vi "Host Main.vi"() -> ()   [LabVIEW 2015]
doc: "This application launches and executes the Tag Bus Data framework configuration for the specified target alias. This is a simple example of the framework API functions, but may also be a suitable starting point for a Host UI or Thick Client that is running a local version of the framework."
uses:
  <vilib>/NI/Module Execution Interface/Engine Runtime/Execution States.ctl
  <vilib>/NI/Module Execution Interface/Engine Runtime/Fault.ctl
  <vilib>/NI/Tag Bus Module Framework/runtime/error classification.ctl
  <vilib>/NI/Current Value Table/DataTypes/Double_Read.vi
  <vilib>/NI/Current Value Table/Type to Enum.vi
  <vilib>/NI/Current Value Table/DataTypes/Double_Type To Enum.vi
  <vilib>/NI/Current Value Table/FGVs/CVT Globals.vi
  <vilib>/NI/Current Value Table/FGVs/Tag Memory.vi
  <vilib>/NI/Current Value Table/Memory Block.vi
  <vilib>/NI/Current Value Table/DataTypes/Double_Memory Block.vi
  <vilib>/NI/Module Execution Interface/Engine Runtime/Engine Runtime Interface.lvclass
  <vilib>/NI/DCAF/Tag Editor Core/Framework Configuration Classes/target runtime/PL_Target Runtime.lvclass
  <vilib>/NI/Tag Bus Module Framework/FPGA manager/FPGA manager.lvlib
  <vilib>/rvi/interface/nirviOpenFPGA/nirviOpenFPGA.xnode
  <vilib>/userdefined/High Color/nirio_resource_hc.ctl
  <vilib>/NI/Tag Bus Module Framework/FPGA manager/methods.ctl
  <vilib>/NI/Tag Bus Module Framework/runtime/TBM module execution interface.lvclass
  <vilib>/NI/Current Value Table/Current Value Table.lvlib
panel:
  out "Temperature":dbl
  in  "configuration file path":path=path "C:/Users/blueuser/Desktop/Hands On/Hands-On_1/myExercises/Temperature Controller/SimulatedSystem.pcfg"
  in  "target alias":string="PC"
  out "engine status":T4(array[cluster])
  in  "stop":bool
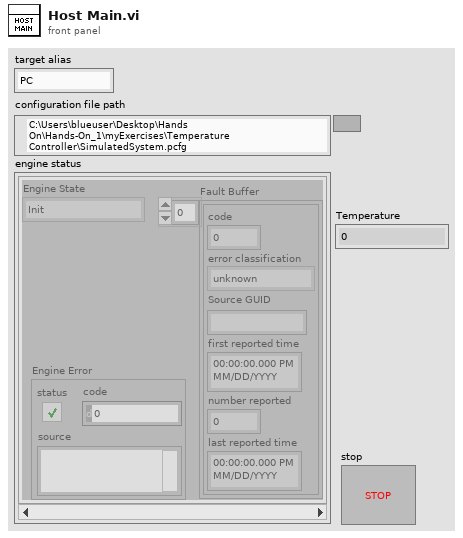
[diagram p1: front panel]
types:
  T1 = typedef "Engine Runtime Interface.lvclass/Execution States.ctl" = enum16{"Init", "Pre-Operational", "Safe-Operational", "Operational", "Stopped"}
  T2 = typedef "Engine Runtime Interface.lvclass/Fault.ctl" = cluster{"code":i32, "error classification":T3, "Source GUID":string, "first reported time":timestamp, "number reported":u32, "last reported time":timestamp}
  T3 = typedef "TBM module execution interface.lvclass/error classification.ctl" = enum16{"unknown", "none", "trivial", "recoverable", "critical"}
  T4 = cluster{"Engine State":T1, "Fault Buffer":T2[], "Engine Error":errorcluster}[]
  T5 = typedef "FPGA manager.lvlib/methods.ctl" = enum16{"initialize bitfile", "cache bitfile", "locate bitfile", "close bitfile", "clear manager"}
  T6 = typedef "nirio_resource_hc.ctl" = tag
  T7 = cluster{"Engine State":T1, "Fault Buffer":T2[], "Engine Error":errorcluster}
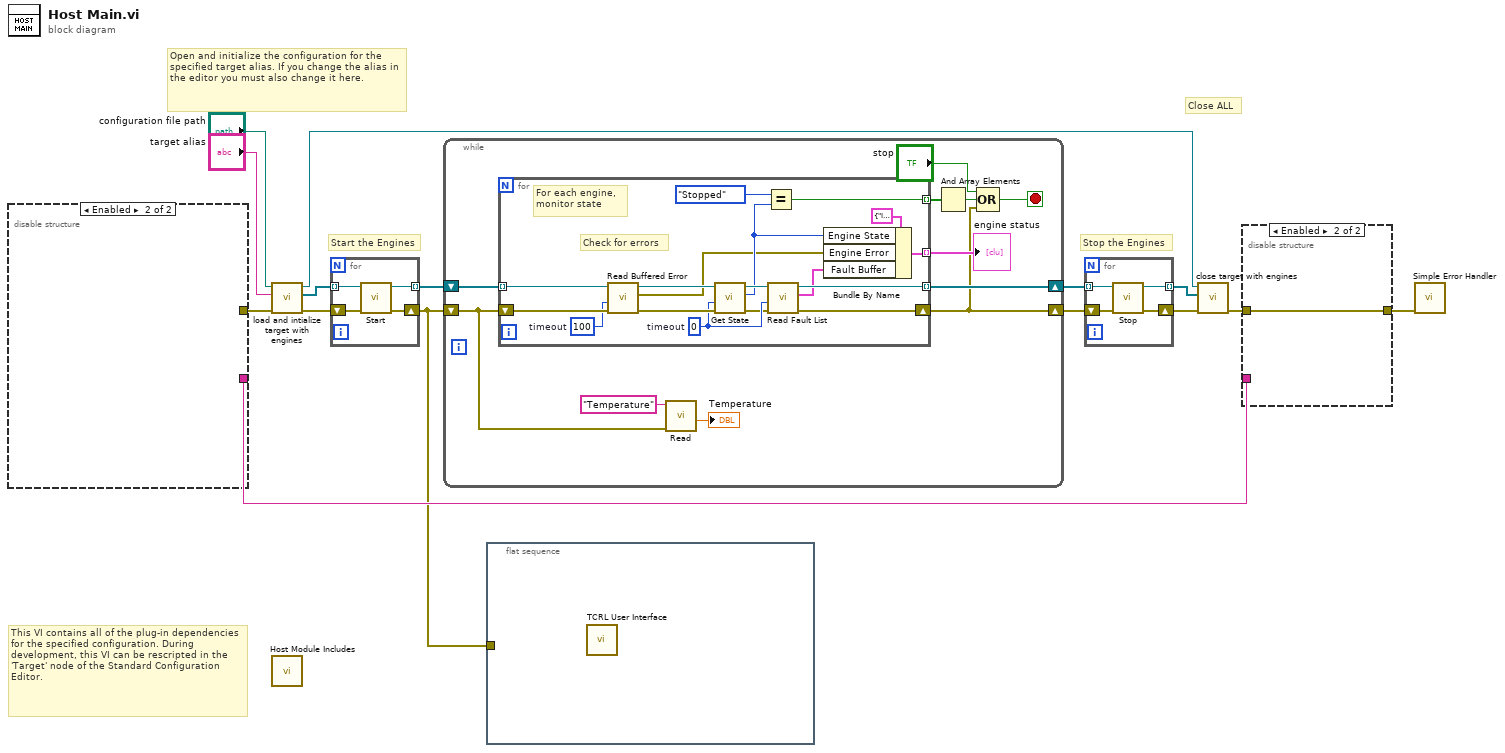
[diagram p0: block diagram]
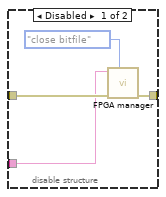
[diagram p2: hidden frame]
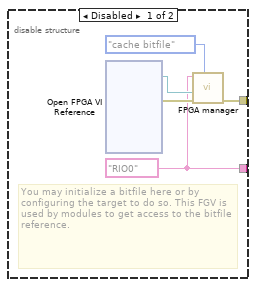
[diagram p3: hidden frame]
diagram:
  # "Start the Engines"
  # "Open and initialize the configuration for the specified target alias. If you change the alias in the editor you must also change it here."
  # "Close ALL"
  # "Stop the Engines"
  # "This VI contains all of the plug-in dependencies for the specified configuration. During development, this VI can be rescripted in the 'Target' node of the Standard Configuration Editor."
  n1 = disable-structure shown="Enabled" {
    disable-tunnel: [w20 _] -> w5
    disable-tunnel: [w16 _] -> w4
    frame Disabled {
      w16 = T6 "RIO0" ("RIO resource")
      # "You may initialize a bitfile here or by configuring the target to do so. This FGV is used by modules to get access to the bitfile reference."
      n2 = xnode "Open FPGA VI Reference"() -> ("FPGA VI Reference Out"=w18:refnum<k20>, "error out"=w19:errorcluster)  [unwired: 2 in]
      n3 = call <vilib>:"FPGA manager.vi"("action"=methods."cache bitfile", "error in"=w19, "bitfile to cache"=w18, "RIO resource"=w16) -> ("error out"=w20:errorcluster)  [unwired: 5 in, 2 out]
    }
    frame Enabled {
    }
  }
  n4 = call <vilib>:"load and intialize target with engines.vi"("error in"=w5, "target alias"="target alias", "file path"="configuration file path") -> ("error out"=w12:errorcluster, "engine runtime interfaces"=w11:refnum<class "Engine Runtime Interface.lvclass">[], "target runtime"=w8:refnum<class "PL_Target Runtime.lvclass">)  [unwired: 6 in]
  n5 = call "Host Module Includes.vi"() -> ()  [unwired: 12 in]
  n6 = for {
    tunnel: [w24] -> w15 mode=indexing
    tunnel: w11 -> [w21] mode=indexing
    shift-right: [w23] -> w2
    shift-left: w12 -> [w22]
    n7 = call-dynamic "Start.vi"("error in"=w22, "Engine Runtime Interface in"=w21) -> ("error out"=w23:errorcluster, "Engine Runtime Interface out"=w24:refnum<class "Engine Runtime Interface.lvclass">)  [unwired: 8 in]
  }
  n8 = while {
    shift-right: [w34] -> w14
    shift-left: w15 -> [w35]
    shift-right: [w28] -> w13
    shift-left: w2 -> [w26]
    stop <- w32 stop-if-true
    n9 = for {
      tunnel: w35 -> [w52] mode=indexing
      tunnel: [w44] -> w34 mode=indexing
      tunnel: [w47] -> w30 mode=indexing
      shift-right: [w43] -> w28
      shift-left: w26 -> [w51]
      tunnel: [w39] -> w31 mode=indexing
      w42 = 0  # timeout
      w46 = 100  # timeout
      # "For each engine, \nmonitor state"
      # "Check for errors"
      n10 = call-dynamic "Read Buffered Error.vi"("error in"=w51, "timeout in ms (0)"=w46, "Engine Runtime Interface in"=w52) -> ("error out"=w49:errorcluster, "Engine Error"=w37:errorcluster, "Engine Runtime Interface out"=w50:refnum<class "Engine Runtime Interface.lvclass">)  [unwired: 6 in]
      n11 = call-dynamic "Get State.vi"("error in"=w49, "timeout (-1)"=w42, "Engine Runtime Interface in"=w50) -> ("error out"=w36:errorcluster, "Engine State"=w41:T1, "Engine Runtime Interface out"=w45:refnum<class "Engine Runtime Interface.lvclass">)  [unwired: 6 in]
      n12 = Equal?(x=Execution_States."Stopped" ("Engine State"), y=w41) -> (x = y?=w47:bool)
      n13 = call-dynamic "Read Fault List.vi"("error in"=w36, "timeout (-1)"=w42, "Engine Runtime Interface in"=w45) -> ("error out"=w43:errorcluster, "faults"=w40:T2[], "Engine Runtime Interface out"=w44:refnum<class "Engine Runtime Interface.lvclass">)  [unwired: 6 in]
      n14 = Bundle By Name(cluster=T7 {"Engine State"=enum."Init", "Fault Buffer"=[], "Engine Error"={"status"=FALSE, "code"=0, "source"=""}}, "Engine State"=w41, "Engine Error"=w37, "Fault Buffer"=w40) -> (w39:T7)
    }
    "engine status" <- w31
    n15 = call-poly <vilib>:"Read.vi"("error in (no error)"=w26, "Tag Name"="Temperature") -> ("Value"=→"Temperature":dbl)  [unwired: 8 in, 1 out]
    n16 = And Array Elements(Boolean array=w30) -> (logical AND=w29:bool)
    n17 = Compound Arithmetic op=OR("stop", w29, w28) -> (w32:bool)
  }
  n18 = flat-sequence {
    tunnel: w2 -> [_]
    frame #0 {
      n19 = call "TCRL User Interface.vi"() -> ()  [unwired: 12 in]
    }
  }
  n20 = for {
    tunnel: w14 -> [w56] mode=indexing
    shift-right: [w53] -> w7
    shift-left: w13 -> [w55]
    tunnel: [w54] -> w9 mode=indexing
    n21 = call-dynamic "Stop.vi"("error in"=w55, "Engine Runtime Interface in"=w56) -> ("error out"=w53:errorcluster, "Engine Runtime Interface out"=w54:refnum<class "Engine Runtime Interface.lvclass">)  [unwired: 8 in]
  }
  n22 = call <vilib>:"close target with engines.vi"("error in"=w7, "Engine Runtime Interfaces"=w9, "Target Runtime"=w8) -> ("error out"=w3:errorcluster)  [unwired: 8 in]
  n23 = disable-structure shown="Enabled" {
    disable-tunnel: [w59 w61] -> w1
    disable-tunnel: w3 -> [w60 w61]
    disable-tunnel: w4 -> [w57 _]
    frame Disabled {
      n24 = call <vilib>:"FPGA manager.vi"("action"=methods."close bitfile", "error in"=w60, "RIO resource"=w57) -> ("error out"=w59:errorcluster)  [unwired: 6 in, 2 out]
    }
    frame Enabled {
    }
  }
  n25 = call <vilib>:"Simple Error Handler.vi"("error in (no error)"=w1) -> ()  [unwired: 4 in, 5 out]
